vi "Eval y=f(x).vi"(4 "formula":string, 5 "end":dbl=1.0 format="%.2f", 6 "start":dbl format="%.2f", 7 "number of points":u32=10) -> (0 "error":i32, 1 "ticks":u32, 2 "Y Values":dbl[](array[numeric]) format="%.2f", 3 "X Values":dbl[](array[numeric]) format="%.2f")   [LabVIEW 2017, in "NI_Gmath.lvlib"]
doc: "Calculates the values of a 1D function given by a <B>formula</B> at equidistant points in an interval."
uses:
  <vilib>/gmath/NI_Gmath.lvlib
panel:
  # "Example:\n\n number of points: 100 \n start: 0.0\n end: 1.0\n formula: sin(t*t)+t"
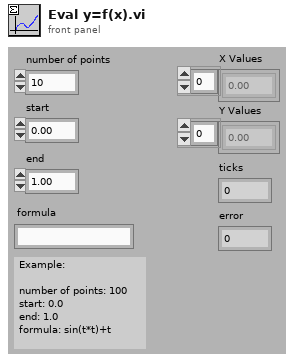
[diagram p1: front panel]
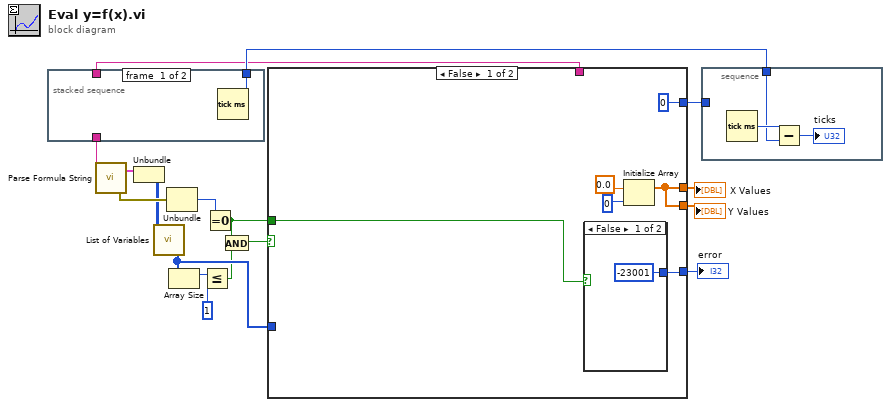
[diagram p0: block diagram]
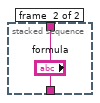
[diagram p2: hidden frame]
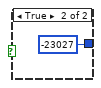
[diagram p3: hidden frame]
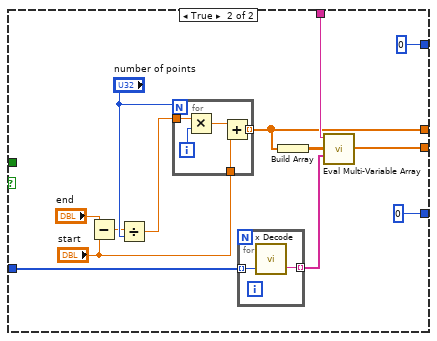
[diagram p4: hidden frame]
diagram:
  n1 = stacked-sequence {
    tunnel: [w18 _] -> w12
    tunnel: [_ "formula"] -> w2
    tunnel: [_ "formula"] -> w1
    frame #0 {
      n2 = Tick Count (ms)() -> (millisecond timer value=w18:u32)
    }
    frame #1 {
    }
  }
  n3 = call <vilib>:"Parse Formula String.vi"("formula"=w1) -> ("error out"=w8:errorcluster, "Parsed Formula"=w4:cluster{"Table":i32[][], "Y Values":dbl[]})  [unwired: 1 in]
  n4 = Unbundle(w4) -> ("Table"=w3:i32[][])  [unwired: 1 out]
  n5 = call <vilib>:"List of Variables.vi"("Table"=w3) -> ("List of variables"=w13:i32[])
  n6 = Unbundle(w8) -> ("code"=w7:i32)  [unwired: 2 out]
  n7 = Array Size(array=w13) -> (size(s)=w15:i32)
  n8 = Less Or Equal?(x=w15, y=1) -> (x <= y?=w5:bool)
  n9 = Equal To 0?(x=w7) -> (x = 0?=w17:bool)
  n10 = And(x=w17, y=w5) -> (x .and. y?=w16:bool)
  n11 = case shown="False" w16 {
    tunnel: w2 -> [_ w40]
    tunnel: w13 -> [_ w39]
    tunnel: [w23 w32] -> w11
    tunnel: [w23 w38] -> w10
    tunnel: [0 0] -> w9
    tunnel: [w21 0] -> w6
    tunnel: w17 -> [w20 _]
    frame False {
      n12 = case shown="False" w20 {
        tunnel: [-23001 -23027] -> w21
        frame False {
        }
        frame True {
        }
      }
      n13 = Initialize Array(0.0, 0) -> (w23:dbl[])
    }
    frame True {
      n14 = Subtract(x="end", y="start") -> (x-y=w33:dbl)
      n15 = Divide(x=w33, y="number of points") -> (x/y=w34:dbl)
      n16 = for {
        N: "number of points" -> [_]
        tunnel: w34 -> [w45]
        tunnel: "start" -> [w42]
        tunnel: [w41] -> w32 mode=indexing
        i -> [w44]
        n17 = Multiply(x=w45, y=w44) -> (x*y=w43:dbl)
        n18 = Add(x=w43, y=w42) -> (x+y=w41:dbl)
      }
      n19 = for {
        tunnel: w39 -> [w47] mode=indexing
        tunnel: [w46] -> w29 mode=indexing
        n20 = call <vilib>:"x Decode.vi"("number"=w47) -> ("x string"=w46:string)  [unwired: 1 in, 1 out]
      }
      n21 = Build Array(w32) -> (w30:dbl[][])
      n22 = call <vilib>:"Eval Multi-Variable Array.vi"("Variables"=w29, "X Values"=w30, "formula"=w40) -> ("Y Values"=w38:dbl[])  [unwired: 1 in, 1 out]
    }
  }
  "error" <- w6
  "X Values" <- w11
  "Y Values" <- w10
  n23 = stacked-sequence {
    tunnel: w12 -> [w48]
    tunnel: w9 -> [_]
    frame #0 {
      n24 = Tick Count (ms)() -> (millisecond timer value=w49:u32)
      n25 = Subtract(x=w49, y=w48) -> (x-y=→"ticks":u32)
    }
  }
